vi "QO_Store_100.vi"(0 "Queue_Name_In":string, 1 "Max_Queue_Size_In":i32=-1, 5 "Time_Out_In_ms (-1)":i32=-1, 7 "Data_In":T1, 11 "Error_In":errorcluster, 13 "Queue_Operation":T2=enum."Flush") -> (3 "Max_Queue_Size_Out":i32=-1, 4 "Queue_Name_Out":string, 8 "Data_Out":T1, 10 "Total_Data":T1[](array[typedef]), 15 "Error_Out":errorcluster)   [LabVIEW 2023]
doc: "Used to transfer data from one vi to another using queue."
uses:
  Controls/Queue_Operation.ctl
  Controls/Generated_data.ctl
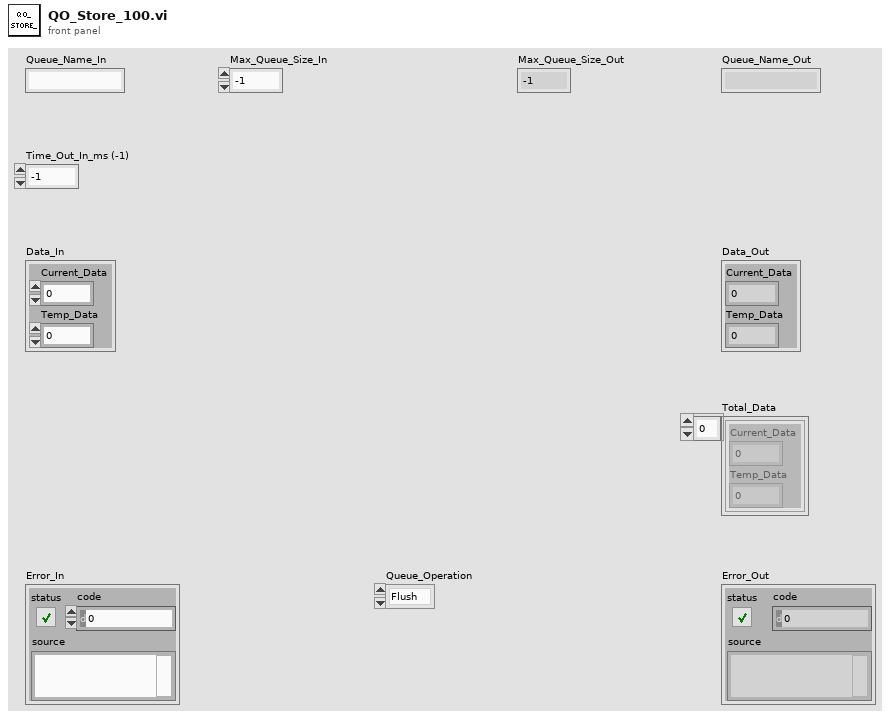
[diagram p1: front panel]
types:
  T1 = typedef "Generated_data.ctl" = cluster{"Current_Data":dbl, "Temp_Data":dbl}
  T2 = typedef "Queue_Operation.ctl" = enum16{"Obtain_Queue", "Enqueue", "Lossy_Enqueue", "Preview", "Queue_Status", "Release_Queue", "Dequeue", "Flush"}
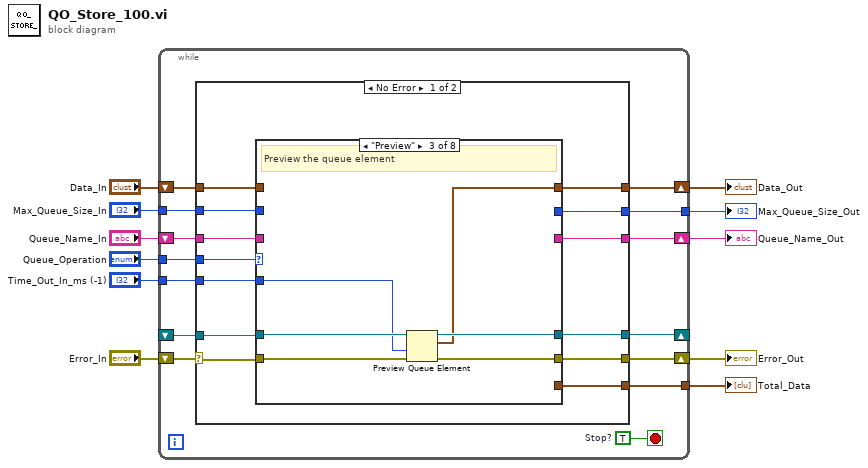
[diagram p0: block diagram]
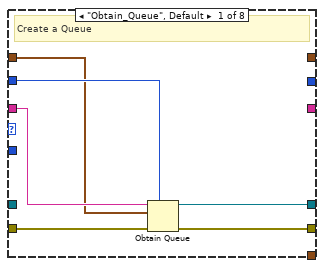
[diagram p2: hidden frame]
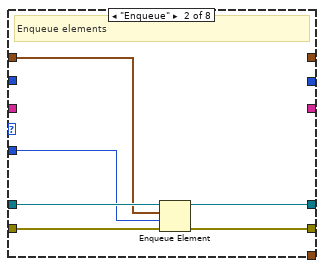
[diagram p3: hidden frame]
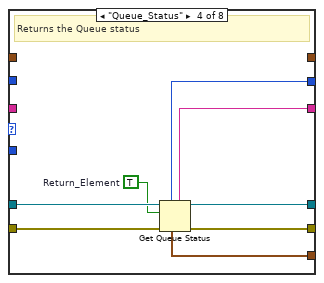
[diagram p4: hidden frame]
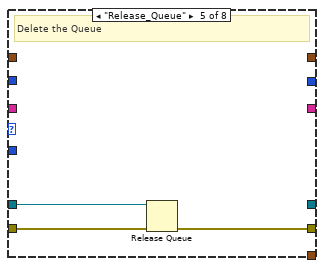
[diagram p5: hidden frame]
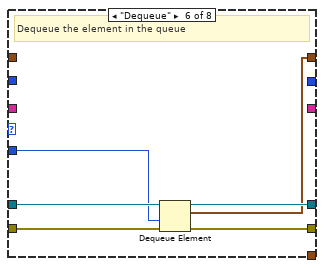
[diagram p6: hidden frame]
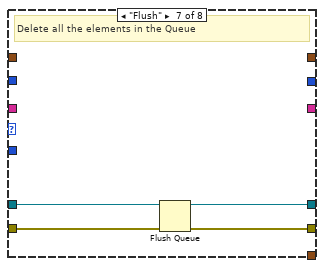
[diagram p7: hidden frame]
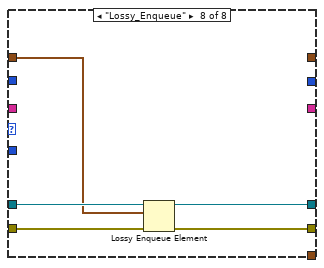
[diagram p8: hidden frame]
diagram:
  n1 = while {
    tunnel: "Max_Queue_Size_In" -> [w25]
    tunnel: "Time_Out_In_ms (-1)" -> [w22]
    tunnel: [w20] -> w6
    tunnel: "Queue_Operation" -> [w17]
    tunnel: [w15] -> w2
    shift-right: [w21] -> w7
    shift-left: "Data_In" -> [w23]
    shift-right: [w19] -> w5
    shift-left: "Queue_Name_In" -> [w16]
    shift-right: [w24] -> w10
    shift-left: "Error_In" -> [w14]
    shift-right: [w18] -> _
    shift-left: _ -> [w13]
    stop <- w12 stop-if-true
    w12 = TRUE  # Stop?
    n2 = case shown="No Error" w14 {
      selector: w14 -> [w27 w83]
      tunnel: w17 -> [w28 _]
      tunnel: w16 -> [w29 _]
      tunnel: w25 -> [w38 _]
      tunnel: [w37 _] -> w18
      tunnel: [w36 w83] -> w24
      tunnel: w23 -> [w30 _]
      tunnel: w22 -> [w35 _]
      tunnel: [w34 _] -> w21
      tunnel: [w33 _] -> w20
      tunnel: [w32 _] -> w19
      tunnel: [w31 _] -> w15
      tunnel: w13 -> [w26 _]
      frame No Error {
        n3 = case shown="\"Preview\"" w28 {
          tunnel: w27 -> [w44 w50 w55 w63 w66 w72 w76 w81]
          tunnel: w29 -> [w42 _ _ _ _ _ _ _]
          tunnel: w38 -> [w41 _ _ _ _ _ _ _]
          tunnel: [w39 w46 w54 w62 _ w71 w75 w80] -> w37
          tunnel: [w43 w49 w53 w61 w65 w69 w74 w79] -> w36
          tunnel: w26 -> [_ w48 w56 w64 w67 w73 w77 w82]
          tunnel: w30 -> [w40 w47 _ _ _ _ _ w78]
          tunnel: w35 -> [_ w45 w52 _ _ w68 _ _]
          tunnel: [_ _ w51 _ _ w70 _ _] -> w34
          tunnel: [_ _ _ w60 _ _ _ _] -> w33
          tunnel: [_ _ _ w59 _ _ _ _] -> w32
          tunnel: [_ _ _ w58 _ _ _ _] -> w31
          frame "Obtain_Queue", Default {
            # "Create a Queue"
            n4 = Obtain Queue(max queue size (-1, unlimited)=w41, name (unnamed)=w42, element data type=w40, error in (no error)=w44) -> (queue out=w39:refnum<queue>, error out=w43:errorcluster)  [unwired: 1 in, 1 out]
          }
          frame "Enqueue" {
            # "Enqueue elements"
            n5 = Enqueue Element(queue=w48, element=w47, timeout in ms (-1)=w45, error in (no error)=w50) -> (queue out=w46:refnum<queue>, error out=w49:errorcluster)  [unwired: 1 out]
          }
          frame "Preview" {
            # "Preview the queue element"
            n6 = Preview Queue Element(queue=w56, timeout in ms (-1)=w52, error in (no error)=w55) -> (queue out=w54:refnum<queue>, element=w51:T1, error out=w53:errorcluster)  [unwired: 1 out]
          }
          frame "Queue_Status" {
            w57 = TRUE  # Return_Element
            # "Returns the Queue status"
            n7 = Get Queue Status(queue=w64, return elements? (F)=w57, error in (no error)=w63) -> (queue out=w62:refnum<queue>, queue name=w59:string, max queue size=w60:i32, error out=w61:errorcluster, elements=w58:T1[])  [unwired: 3 out]
          }
          frame "Release_Queue" {
            # "Delete the Queue"
            n8 = Release Queue(queue=w67, error in (no error)=w66) -> (error out=w65:errorcluster)  [unwired: 1 in, 2 out]
          }
          frame "Dequeue" {
            # "Dequeue the element in the queue"
            n9 = Dequeue Element(queue=w73, timeout in ms (-1)=w68, error in (no error)=w72) -> (queue out=w71:refnum<queue>, element=w70:T1, error out=w69:errorcluster)  [unwired: 1 out]
          }
          frame "Flush" {
            # "Delete all the elements in the Queue"
            n10 = Flush Queue(queue=w77, error in (no error)=w76) -> (queue out=w75:refnum<queue>, error out=w74:errorcluster)  [unwired: 1 out]
          }
          frame "Lossy_Enqueue" {
            n11 = Lossy Enqueue Element(queue=w82, element=w78, error in (no error)=w81) -> (queue out=w80:refnum<queue>, error out=w79:errorcluster)  [unwired: 2 out]
          }
        }
      }
      frame Error {
      }
    }
  }
  "Error_Out" <- w10
  "Data_Out" <- w7
  "Max_Queue_Size_Out" <- w6
  "Queue_Name_Out" <- w5
  "Total_Data" <- w2
